vi "Copy_SourceItem.vi"(7 "referencedNonLVTypeMembers in":T1[](array[typedef]), 8 "error in (no error)":errorcluster, 10 "AB_Build.lvclass":refnum<class "AB_Build.lvclass">, 11 "AB_Source_Container in":refnum<class "AB_Source_Container.lvclass">) -> (0 "error out":errorcluster, 1 "newFileFlags":T2, 2 "newFileInfo":T3, 3 "AB_Source_Container out":refnum<class "AB_Source_Container.lvclass">, 5 "referencedNonLVTypeMembers out":T1[](array[typedef]))   [LabVIEW 2020, in "AB_Source_Container.lvclass"]
uses:
  <vilib>/AppBuilder/AB_Classes/Source/Container/AB_Source_Container.lvclass
  <vilib>/AppBuilder/AB_Classes/Build/AB_Build.lvclass
  <vilib>/AppBuilder/Engine/AB_Engine_New_File_Info.ctl
  <vilib>/AppBuilder/Engine/AB_Engine_New_File_Flags.ctl
  <vilib>/AppBuilder/AB_Source_Referenced_Libray_Files.ctl
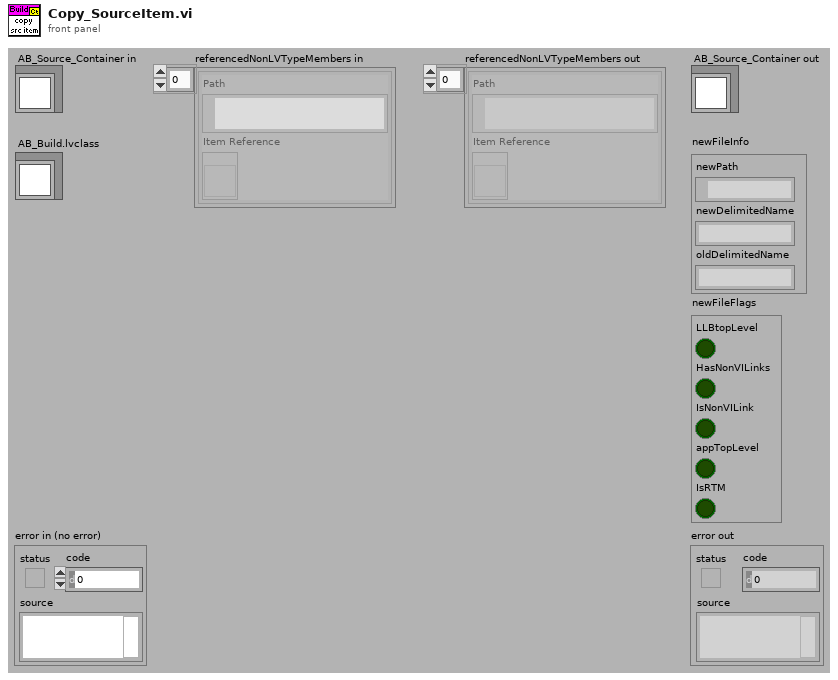
[diagram p1: front panel]
types:
  T1 = typedef "AB_Source_Referenced_Libray_Files.ctl" = cluster{"Path":path, "Item Reference":refnum<vi>}
  T2 = typedef "AB_Engine_New_File_Flags.ctl" = cluster{"LLBtopLevel":bool, "HasNonVILinks":bool, "IsNonVILink":bool, "appTopLevel":bool, "IsRTM":bool}
  T3 = typedef "AB_Engine_New_File_Info.ctl" = cluster{"newPath":path, "newDelimitedName":string, "oldDelimitedName":string}
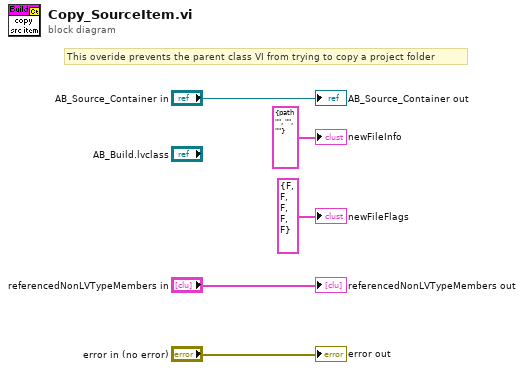
[diagram p0: block diagram]
diagram:
  # "This overide prevents the parent class VI from trying to copy a project folder"
  "error out" <- "error in (no error)"
  "AB_Source_Container out" <- "AB_Source_Container in"
  "newFileInfo" <- T3 {"newPath"=path "", "newDelimitedName"="", "oldDelimitedName"=""} ("newFileInfo")
  "newFileFlags" <- T2 {"LLBtopLevel"=FALSE, "HasNonVILinks"=FALSE, "IsNonVILink"=FALSE, "appTopLevel"=FALSE, "IsRTM"=FALSE} ("newFileFlags")
  "referencedNonLVTypeMembers out" <- "referencedNonLVTypeMembers in"
